vi "Wait For AO Queue.vi"(8 "error in (no error)":errorcluster, 10 "timeout (ms)":i32=5000) -> (0 "error out":errorcluster={"status"=TRUE, "code"=555, "source"="Timed out waiting for Signal Bank."})   [LabVIEW 2020]
uses:
  PXI Globals.vi
panel:
  out "Elapsed time (ms)":u32
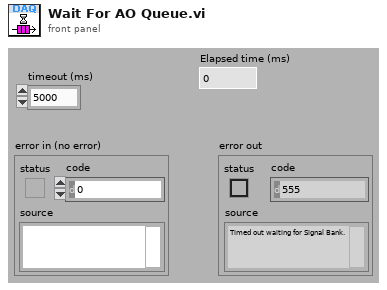
[diagram p1: front panel]
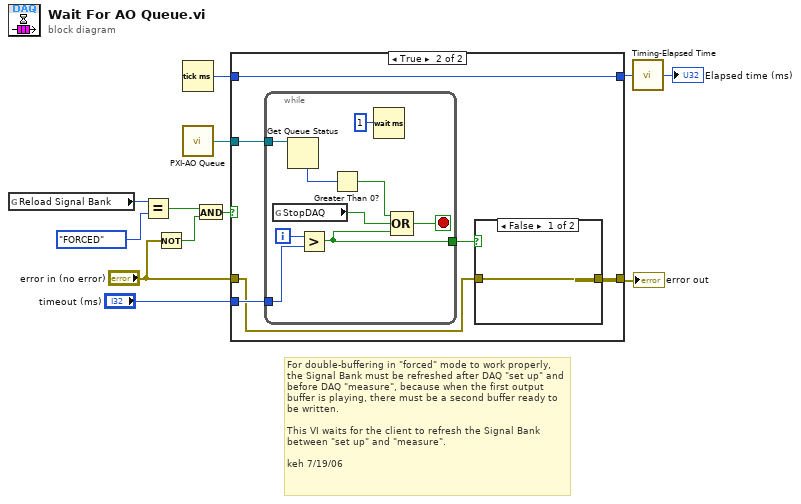
[diagram p0: block diagram]
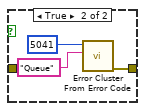
[diagram p3: hidden frame]
diagram:
  # "For double-buffering in \"forced\" mode to work properly, the Signal Bank must be refreshed after DAQ \"set up\" and before DAQ \"measure\", because when the first output buffer is playing, there must be a second buffer ready to be written. \n\nThis VI waits for the client to refresh the Signal Bank between \"set up\" and \"measure\".\n\nkeh 7/19/06"
  n1 = global read "PXI Globals.vi" "Reload Signal Bank"() -> (w12:enum32{"OFF", "ENABLED", "FORCED"})
  n2 = Equal?(x=w12, y=enum16{"OFF", "ENABLED", "FORCED"}."FORCED") -> (x = y?=w6:bool)
  n3 = Not(x="error in (no error)") -> (.not. x?=w9:bool)
  n4 = Tick Count (ms)() -> (millisecond timer value=w4:u32)
  n5 = call "PXI-AO Queue.vi"() -> ("Queue"=w1:refnum<queue>)  [unwired: 15 in]
  n6 = And(x=w6, y=w9) -> (x .and. y?=w8:bool)
  n7 = case shown="True" w8 {
    tunnel: "error in (no error)" -> [w13 w16]
    tunnel: [w13 w18] -> w10
    tunnel: "timeout (ms)" -> [_ w17]
    tunnel: w4 -> [_ w15]
    tunnel: [_ w15] -> w3
    tunnel: w1 -> [_ w14]
    frame False {
    }
    frame True {
      n8 = while {
        tunnel: w17 -> [w26]
        tunnel: [w24] -> w19
        tunnel: w14 -> [w22]
        i -> [w27]
        stop <- w28 stop-if-true
        n9 = global read "PXI Globals.vi" "StopDAQ"() -> (w25:bool)
        n10 = Get Queue Status(queue=w22) -> (# elements in queue=w21:i32)  [unwired: 2 in, 7 out]
        n11 = Greater?(x=w27, y=w26) -> (0:w24:bool)
        n12 = Greater Than 0?(x=w21) -> (x > 0?=w20:bool)
        n13 = Wait (ms)(milliseconds to wait=1) -> ()  [unwired: 1 out]
        n14 = Compound Arithmetic op=OR(w20, w25, w24) -> (w28:bool)
      }
      n15 = case shown="False" w19 {
        tunnel: w16 -> [w29 _]
        tunnel: [w29 w32] -> w18
        frame False {
        }
        frame True {
          n16 = call <vilib>:"Error Cluster From Error Code.vi"("error message (\"\")"="Queue" ("error message (\"\")"), "error code (0)"=5041) -> ("error out"=w32:errorcluster)  [unwired: 7 in]
        }
      }
    }
  }
  "error out" <- w10
  n17 = call "Timing-Elapsed Time.vi"("Start time (ms)"=w3) -> ("Elapsed time (ms)"=→"Elapsed time (ms)":u32)  [unwired: 4 in]
